vi "main.vi"   [LabVIEW 2016]
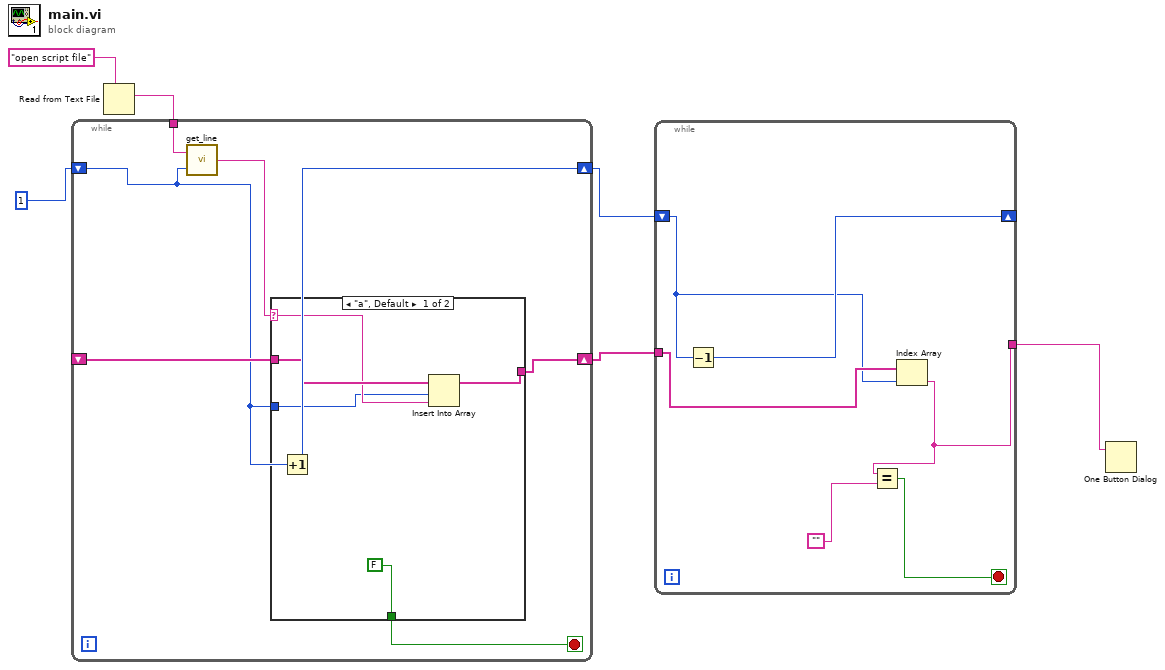
[diagram p0: block diagram]
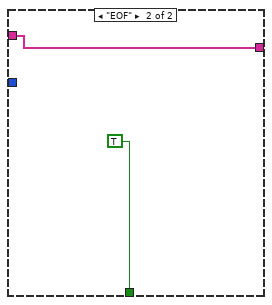
[diagram p2: hidden frame]
diagram:
  n1 = Read from Text File(prompt (Open existing file)="open script file") -> (text=w5:string)  [unwired: 3 in, 3 out]
  n2 = while {
    tunnel: w5 -> [w13]
    shift-right: [w12] -> w2
    shift-left: 1 -> [w7]
    shift-right: [w9] -> w3
    shift-left: _ -> [w8]
    stop <- w10 stop-if-true
    n3 = call "get_line.vi"("line index"=w7, "multi-line string"=w13) -> ("output string"=w11:string)
    n4 = case shown="\"a\", Default" w11 {
      selector: w11 -> [w15 _]
      tunnel: [FALSE TRUE] -> w10
      tunnel: [w17 w19] -> w9
      tunnel: w8 -> [w16 w19]
      tunnel: w7 -> [w14 _]
      frame "a", Default {
        n5 = Insert Into Array(array=w16, index=w14, new element=w15) -> (w17:string[])
      }
      frame "EOF" {
      }
    }
    n6 = Increment(x=w7) -> (x+1=w12:i32)
  }
  n7 = while {
    shift-right: [w26] -> _
    shift-left: w2 -> [w24]
    tunnel: w3 -> [w25]
    tunnel: [w21] -> w1
    stop <- w22 stop-if-true
    n8 = Decrement(x=w24) -> (x-1=w26:i32)
    n9 = Index Array(array=w25, index=w24) -> (element=w21:string)
    n10 = Equal?(x=w21, y="") -> (x = y?=w22:bool)
  }
  n11 = One Button Dialog(message=w1) -> ()  [unwired: 1 in, 1 out]
